vi "tdms_properties_from_metadat.vi"(8 "error in (no error)":errorcluster, 9 "wiring":string[][](array[string])=[["    Electrode 1", " Lockin 1", " ", " KH 1: Ground", " 10x", " Open"], ["    Electrode 2", " Lockin 2", " ", " KH 2: Ground", " 10x", " Open"], ["    Electrode 3", " Lockin 3", " I+", " KH 3: Differential", " 10x", " 50k Ohms"], ["    Electrode 4", " Lockin 4", " I-", " KH 4: Differential", " 10x", " 50k Ohms"], ["    Electrode 5", " Lockin 5", " V1-", " KH 5: SE+ (-gnd)", " 10x", " Open"], ["    Electrode 27", " Lockin 7", " Vbg", " KH 7: Differential", " 10x", " 50k Ohms"], ["    Electrode 28", " Lockin 8", " V1+", " KH 8: SE+ (-gnd)", " 10x", " Open"]], 10 "data":T1, 11 "Experiment Parameters From 1st ITX":T2) -> (0 "error out":errorcluster, 2 "property values":variant[](array[variant]), 3 "property names":string[](array[string]))   [LabVIEW 2016]
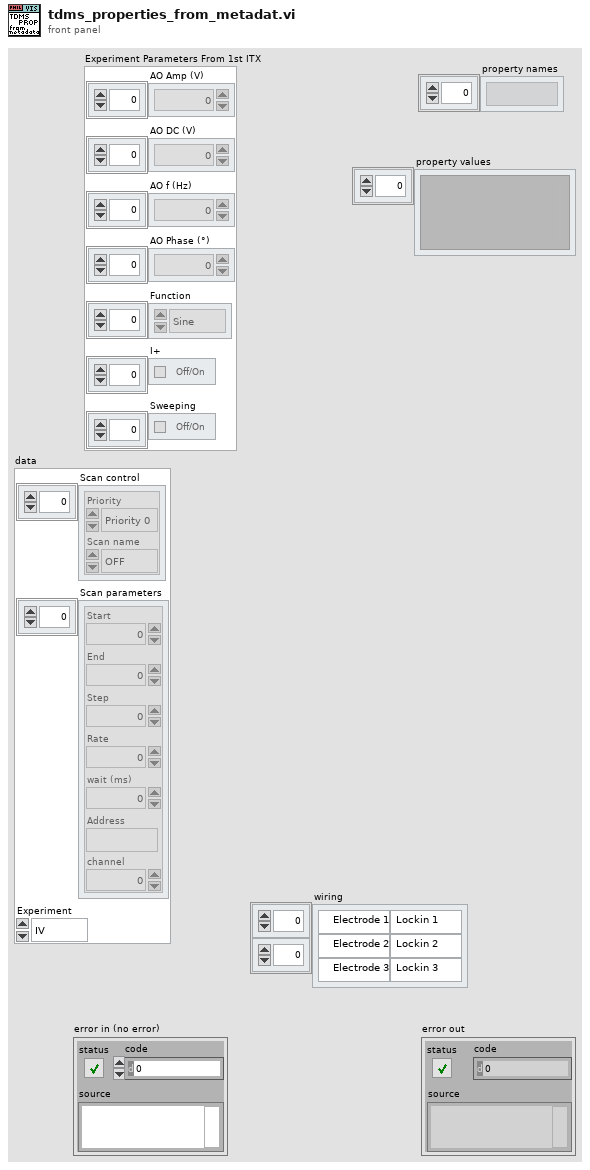
[diagram p1: front panel]
types:
  T1 = cluster{"Scan control":cluster{"Priority":enum16{"Priority 0", "Priority 1", "Priority 2", "Priority 3", "Priority 4", "Priority 5"}, "Scan name":enum16{"OFF", "DSA_Vsg2", "DSA_Vsg3", "DSA_Vbg", "DSA_Vsg1", "DSA_freq", "DSA_Vamp", "time", "Lockin Amplitude", "Lockin Frequency", "Lockin Bias", "Delay", "Strain", "DAQ Bias", "Magnet Field", "Temperature", "MW f1", "MW f2", "MW Amplitude1", "MW Amplitude2"}}[], "Scan parameters":cluster{"Start":dbl, "End":dbl, "Step":dbl, "Rate":dbl, "wait (ms)":u32, "Address":string, "channel":i32}[], "Experiment":enum16{"IV", "IV_Fast", "IV_Sweep", "THz_DelayLine", "Lockin_Vsg", "Lockin_Sweep", "Lockin_Time", "AI WFM time", "Lockin (experimental)"}}
  T2 = cluster{"AO Amp (V)":dbl[], "AO DC (V)":dbl[], "AO f (Hz)":dbl[], "AO Phase (°)":dbl[], "Function":enum16{"Sine", "Triangle", "Square", "Sawtooth"}[], "I+":bool[], "Sweeping":bool[]}
  T3 = cluster{"Priority":enum16{"Priority 0", "Priority 1", "Priority 2", "Priority 3", "Priority 4", "Priority 5"}, "Scan name":enum16{"OFF", "DSA_Vsg2", "DSA_Vsg3", "DSA_Vbg", "DSA_Vsg1", "DSA_freq", "DSA_Vamp", "time", "Lockin Amplitude", "Lockin Frequency", "Lockin Bias", "Delay", "Strain", "DAQ Bias", "Magnet Field", "Temperature", "MW f1", "MW f2", "MW Amplitude1", "MW Amplitude2"}}[]
  T4 = cluster{"Start":dbl, "End":dbl, "Step":dbl, "Rate":dbl, "wait (ms)":u32, "Address":string, "channel":i32}[]
  T5 = enum16{"IV", "IV_Fast", "IV_Sweep", "THz_DelayLine", "Lockin_Vsg", "Lockin_Sweep", "Lockin_Time", "AI WFM time", "Lockin (experimental)"}
  T6 = enum16{"Sine", "Triangle", "Square", "Sawtooth"}[]
  T7 = enum16{"Priority 0", "Priority 1", "Priority 2", "Priority 3", "Priority 4", "Priority 5"}
  T8 = enum16{"OFF", "DSA_Vsg2", "DSA_Vsg3", "DSA_Vbg", "DSA_Vsg1", "DSA_freq", "DSA_Vamp", "time", "Lockin Amplitude", "Lockin Frequency", "Lockin Bias", "Delay", "Strain", "DAQ Bias", "Magnet Field", "Temperature", "MW f1", "MW f2", "MW Amplitude1", "MW Amplitude2"}
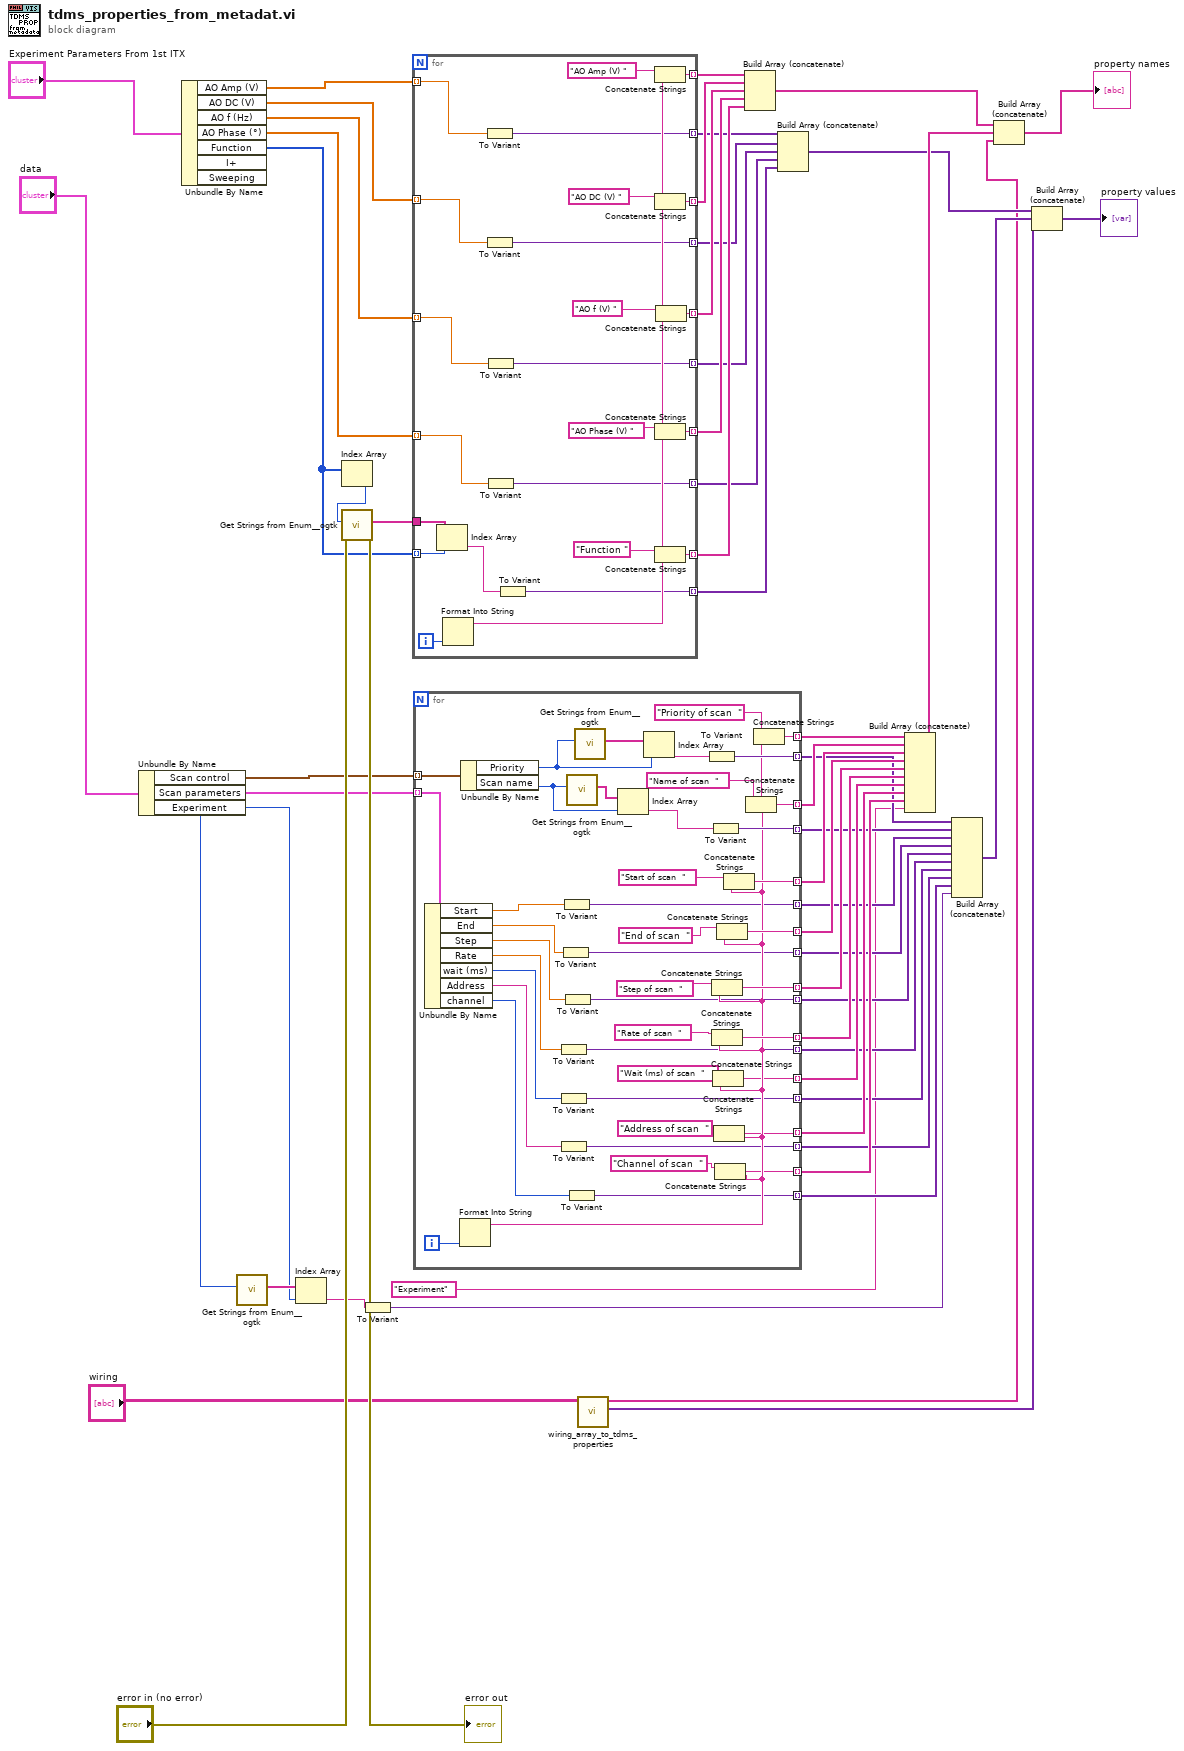
[diagram p0: block diagram]
diagram:
  n1 = Unbundle By Name("data") -> ("Scan control"=w35:T3, "Scan parameters"=w34:T4, "Experiment"=w32:T5)
  n2 = Unbundle By Name("Experiment Parameters From 1st ITX") -> ("AO Amp (V)"=w54:dbl[], "AO DC (V)"=w53:dbl[], "AO f (Hz)"=w52:dbl[], "AO Phase (°)"=w51:dbl[], "Function"=w37:T6)  [unwired: 2 out]
  n3 = call <userlib>:"Get Strings from Enum__ogtk.vi"("Enum"=w32) -> ("Enum Strings"=w33:string[])  [unwired: 7 in, 3 out]
  n4 = Index Array(array=w33, index=w32) -> (element=w10:string)
  n5 = Index Array(array=w37) -> (element=w36:enum16{"Sine", "Triangle", "Square", "Sawtooth"})  [unwired: 1 in]
  n6 = call <userlib>:"Get Strings from Enum__ogtk.vi"("error in (no error)"="error in (no error)", "Enum"=w36) -> ("error out"=→"error out":errorcluster, "Enum Strings"=w45:string[])  [unwired: 6 in, 2 out]
  n7 = To Variant(anything=w10) -> (Variant=w9:variant)
  n8 = for {
    tunnel: w54 -> [w67] mode=indexing
    tunnel: w53 -> [w66] mode=indexing
    tunnel: w52 -> [w64] mode=indexing
    tunnel: w51 -> [w65] mode=indexing
    tunnel: w37 -> [w62] mode=indexing
    tunnel: [w72] -> w50 mode=indexing
    tunnel: [w71] -> w49 mode=indexing
    tunnel: [w70] -> w48 mode=indexing
    tunnel: [w69] -> w47 mode=indexing
    tunnel: [w68] -> w46 mode=indexing
    tunnel: w45 -> [w63]
    tunnel: [w60] -> w40 mode=indexing
    tunnel: [w59] -> w41 mode=indexing
    tunnel: [w58] -> w42 mode=indexing
    tunnel: [w57] -> w43 mode=indexing
    tunnel: [w56] -> w44 mode=indexing
    i -> [w79]
    n9 = Index Array(array=w63, index=w62) -> (element=w61:string)
    n10 = Format Into String(w79) -> (resulting string=w77:string)  [unwired: 3 in, 1 out]
    n11 = To Variant(anything=w67) -> (Variant=w56:variant)
    n12 = To Variant(anything=w66) -> (Variant=w57:variant)
    n13 = To Variant(anything=w64) -> (Variant=w58:variant)
    n14 = To Variant(anything=w65) -> (Variant=w59:variant)
    n15 = To Variant(anything=w61) -> (Variant=w60:variant)
    n16 = Concatenate Strings("AO Amp (V) ", w77) -> (w72:string)
    n17 = Concatenate Strings("AO DC (V) ", w77) -> (w71:string)
    n18 = Concatenate Strings("AO Phase (V) ", w77) -> (w69:string)
    n19 = Concatenate Strings("Function ", w77) -> (w68:string)
    n20 = Concatenate Strings("AO f (V) ", w77) -> (w70:string)
  }
  n21 = for {
    tunnel: w35 -> [w123] mode=indexing
    tunnel: w34 -> [w122] mode=indexing
    tunnel: [w116] -> w19 mode=indexing
    tunnel: [w115] -> w28 mode=indexing
    tunnel: [w113] -> w27 mode=indexing
    tunnel: [w109] -> w18 mode=indexing
    tunnel: [w104] -> w26 mode=indexing
    tunnel: [w103] -> w25 mode=indexing
    tunnel: [w102] -> w24 mode=indexing
    tunnel: [w101] -> w23 mode=indexing
    tunnel: [w89] -> w22 mode=indexing
    tunnel: [w88] -> w21 mode=indexing
    tunnel: [w87] -> w20 mode=indexing
    tunnel: [w86] -> w17 mode=indexing
    tunnel: [w85] -> w16 mode=indexing
    tunnel: [w84] -> w15 mode=indexing
    tunnel: [w83] -> w14 mode=indexing
    tunnel: [w82] -> w13 mode=indexing
    tunnel: [w81] -> w12 mode=indexing
    tunnel: [w80] -> w11 mode=indexing
    i -> [w119]
    n22 = Unbundle By Name(w122) -> ("Start"=w100:dbl, "End"=w99:dbl, "Step"=w98:dbl, "Rate"=w97:dbl, "wait (ms)"=w96:u32, "Address"=w94:string, "channel"=w95:i32)
    n23 = Format Into String(w119) -> (resulting string=w90:string)  [unwired: 3 in, 1 out]
    n24 = Unbundle By Name(w123) -> ("Priority"=w120:T7, "Scan name"=w111:T8)
    n25 = To Variant(anything=w97) -> (Variant=w83:variant)
    n26 = To Variant(anything=w96) -> (Variant=w82:variant)
    n27 = To Variant(anything=w94) -> (Variant=w81:variant)
    n28 = To Variant(anything=w99) -> (Variant=w85:variant)
    n29 = To Variant(anything=w100) -> (Variant=w86:variant)
    n30 = To Variant(anything=w98) -> (Variant=w84:variant)
    n31 = call <userlib>:"Get Strings from Enum__ogtk.vi"("Enum"=w111) -> ("Enum Strings"=w112:string[])  [unwired: 7 in, 3 out]
    n32 = To Variant(anything=w95) -> (Variant=w80:variant)
    n33 = call <userlib>:"Get Strings from Enum__ogtk.vi"("Enum"=w120) -> ("Enum Strings"=w121:string[])  [unwired: 7 in, 3 out]
    n34 = Index Array(array=w112, index=w111) -> (element=w110:string)
    n35 = Index Array(array=w121, index=w120) -> (element=w117:string)
    n36 = To Variant(anything=w117) -> (Variant=w116:variant)
    n37 = To Variant(anything=w110) -> (Variant=w109:variant)
    n38 = Concatenate Strings("Step of scan  ", w90) -> (w102:string)
    n39 = Concatenate Strings("Rate of scan  ", w90) -> (w101:string)
    n40 = Concatenate Strings("Wait (ms) of scan  ", w90) -> (w89:string)
    n41 = Concatenate Strings("Address of scan  ", w90) -> (w88:string)
    n42 = Concatenate Strings("Channel of scan  ", w90) -> (w87:string)
    n43 = Concatenate Strings("End of scan  ", w90) -> (w103:string)
    n44 = Concatenate Strings("Start of scan  ", w90) -> (w104:string)
    n45 = Concatenate Strings("Name of scan  ", w90) -> (w113:string)
    n46 = Concatenate Strings("Priority of scan  ", w90) -> (w115:string)
  }
  n47 = call "wiring_array_to_tdms_properties.vi"("wiring"="wiring") -> ("property values"=w3:variant[], "property names"=w2:string[])  [unwired: 9 in]
  n48 = Build Array (concatenate)(w50, w49, w48, w47, w46) -> (w31:string[])
  n49 = Build Array (concatenate)(w44, w43, w42, w41, w40) -> (w6:variant[])
  n50 = Build Array (concatenate)(w28, w27, w26, w25, w24, w23, w22, w21, w20, "Experiment") -> (w7:string[])
  n51 = Build Array (concatenate)(w19, w18, w17, w16, w15, w14, w13, w12, w11, w9) -> (w4:variant[])
  n52 = Build Array (concatenate)(w31, w7, w2) -> (→"property names":string[])
  n53 = Build Array (concatenate)(w6, w4, w3) -> (→"property values":variant[])
